vi "Find All Async Methods Actors In Project.vi"(8 "error in (no error)":errorcluster, 9 "Include Dependencies?":bool, 11 "Project Item in":refnum<vi>) -> (0 "error out":errorcluster, 1 "Async Methods Acotrs Paths":path[](array[path]), 2 "Async Methods Acotrs Names":string[](array[string]), 3 "Project Item out":refnum<vi>)   [LabVIEW 2023, in "Add Async Methods Actor.lvlib" / "Live Store.lvclass"]
doc: "Finds all actors in the project\n\nAuthor: Derek Trepanier\nCopyright: MGI 2015"
uses:
  Live Store.lvclass
  Live Store.lvclass/Live Store.ctl
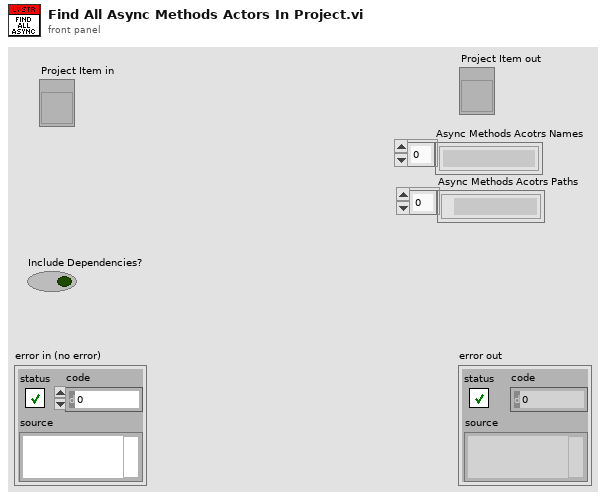
[diagram p1: front panel]
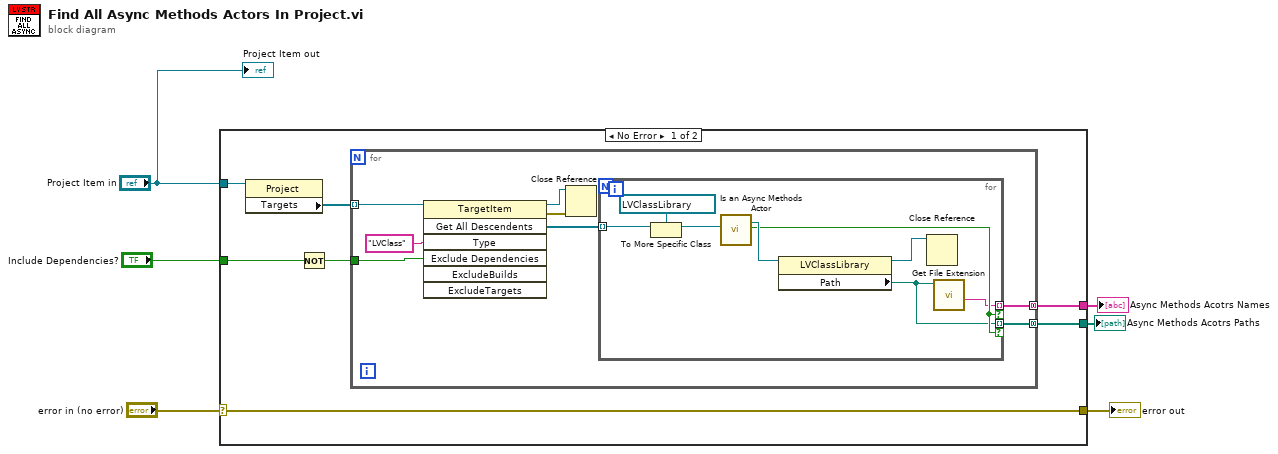
[diagram p0: block diagram]
diagram:
  n1 = case shown="No Error" "error in (no error)" {
    selector: "error in (no error)" -> [w13 w30]
    tunnel: [w13 w30] -> w5
    tunnel: "Include Dependencies?" -> [w11 _]
    tunnel: "Project Item in" -> [w9 _]
    tunnel: [w8 _] -> w2
    tunnel: [w7 _] -> w1
    frame No Error {
      n2 = property class="Project"(reference=w9) -> ("Targets"=w12:refnum<vi>[])  [unwired: 1 in, 2 out]
      n3 = Not(x=w11) -> (.not. x?=w10:bool)
      n4 = for {
        tunnel: w12 -> [w21] mode=indexing
        tunnel: w10 -> [w19]
        tunnel: [w15] -> w8 mode=concatenating
        tunnel: [w14] -> w7 mode=concatenating
        n5 = invoke class="TargetItem" method="Get All Descendents"(reference=w21, "Type"="LVClass", "Exclude Dependencies"=w19) -> (reference out=w16:refnum<vi>, error out=w17:errorcluster, "All Descendents"=w18:refnum<vi>[])  [unwired: 4 in, 4 out]
        n6 = Close Reference(reference=w16, error in (no error)=w17) -> ()  [unwired: 1 out]
        n7 = for {
          tunnel: w18 -> [w29] mode=indexing
          tunnel: [w22] -> w15 mode=indexing if=w25
          tunnel: [w23] -> w14 mode=indexing if=w25
          n8 = To More Specific Class(target class=refnum<vi> refnum ("reference out"), reference=w29) -> (specific class reference=w27:refnum<vi>)  [unwired: 1 in, 1 out]
          n9 = call "Is an Async Methods Actor.vi"("Class in"=w27) -> ("Class out"=w26:refnum<vi>, "Is Async Method Actor?"=w25:bool)  [unwired: 16 in, 1 out]
          n10 = property class="LVClassLibrary"(reference=w26) -> (reference out=w24:refnum<vi>, "Path"=w23:path)  [unwired: 1 in, 1 out]
          n11 = Close Reference(reference=w24) -> ()  [unwired: 1 in, 1 out]
          n12 = call <vilib>:"Get File Extension.vi"("file"=w23) -> ("filename without extension"=w22:string)  [unwired: 6 in, 4 out]
        }
      }
    }
    frame Error {
    }
  }
  "error out" <- w5
  "Async Methods Acotrs Names" <- w2
  "Async Methods Acotrs Paths" <- w1
  "Project Item out" <- "Project Item in"
